vi "STAGE+mono+counter_edit3.vi"() -> ()   [LabVIEW 2017]
panel:
  out "XY Graph":cluster{"Y":dbl[], "Y":dbl[]}[](graph)
  in  "Integrating time, 10^-7 sec":dbl=10000000.0
  out "Timeout 2":bool
  in  "scan from":i32=2600
  in  "scan to":i32=4000
  in  "?":bool
  in  "Exit Labview":bool
  in  "step size":dbl=10.0 min=0.0
  in  "?":bool
  out "Spectrum":waveform(dbl)(graph)
  out "Counts":i32
  in  "value (0)":dbl=-9.0
  out "Current WL Wavelength  2":u16 caption="Current Wavelength"
  out "Grt# 2":u8=1 min=1 max=3 step=1
  out "Blaze (nm)":u32=300
  out "Groove/mm":u32=1200
  in  "?":bool
  in  "Channel B Input":u16(ring)=2 items=["Input 1"=1, "Input 2"=2]
  in  "Trigger mode":u16(ring) items=["10 MHz"=0, "Input 2"=2, "Input T"=3]
  out "Current WL Wavelength":u16 caption="Current Wavelength"
  in  "Integrating time, 10^-7 sec":dbl=10000000.0
  in  "gate A mode (CW:0)":i16(slide) scale=0.0..2.0 scale format="%.2f"
  in  "Channel A Input":u16(ring)=1 items=["10 MHz", "Input 1"]
  in  "Time between measurements\n at one point (s)/Dwell Time":dbl=0.002 min=0.002 max=60.0 step=0.001
  in  "Number of Measurements\n to take at one point/ Number of Periods":u16=1 min=1 max=2000 step=1
  in  "Count Mode":u16(ring) items=["A,B for Preset T", "A-B for Preset T", "A+B for Preset T", "A for Preset B"]
  in  "GPIB address":string="23"
  out "Timeout":bool
  out "Serial":u32=12345
  out "Grt#":u8=1 min=1 max=3 step=1
  out "Blaze (nm)":u32=300
  out "Groove/mm":u32=1200
  out "time delay":u32=450000 min=1
  out "Mono port":T1(ring)
  in  "Get position":bool
  out "Position status":dbl format="%.3f"
  in  "Target position":dbl format="%.3f"
  in  "Move":bool
  in  "Motor OFF":bool
  in  "Motor ON":bool
  in  "Step Size [um]":i32=10
  in  "Axis":i32=1
  in  "Rep Rate [Hz]":dbl=500.0
  out "Shots":dbl
  in  "Averaging Time [s]":dbl=0.1
  out "Current Point":i32
  out "Slide":i32(slide) scale=0.0..100.0
  out "Current Position [mm]":dbl
  in  "Axis initial position [mm]":dbl
  out "Axis final Position [mm]":dbl
  in  "Data Points (100 default)":i32=100
  in  "Collect Data!":bool
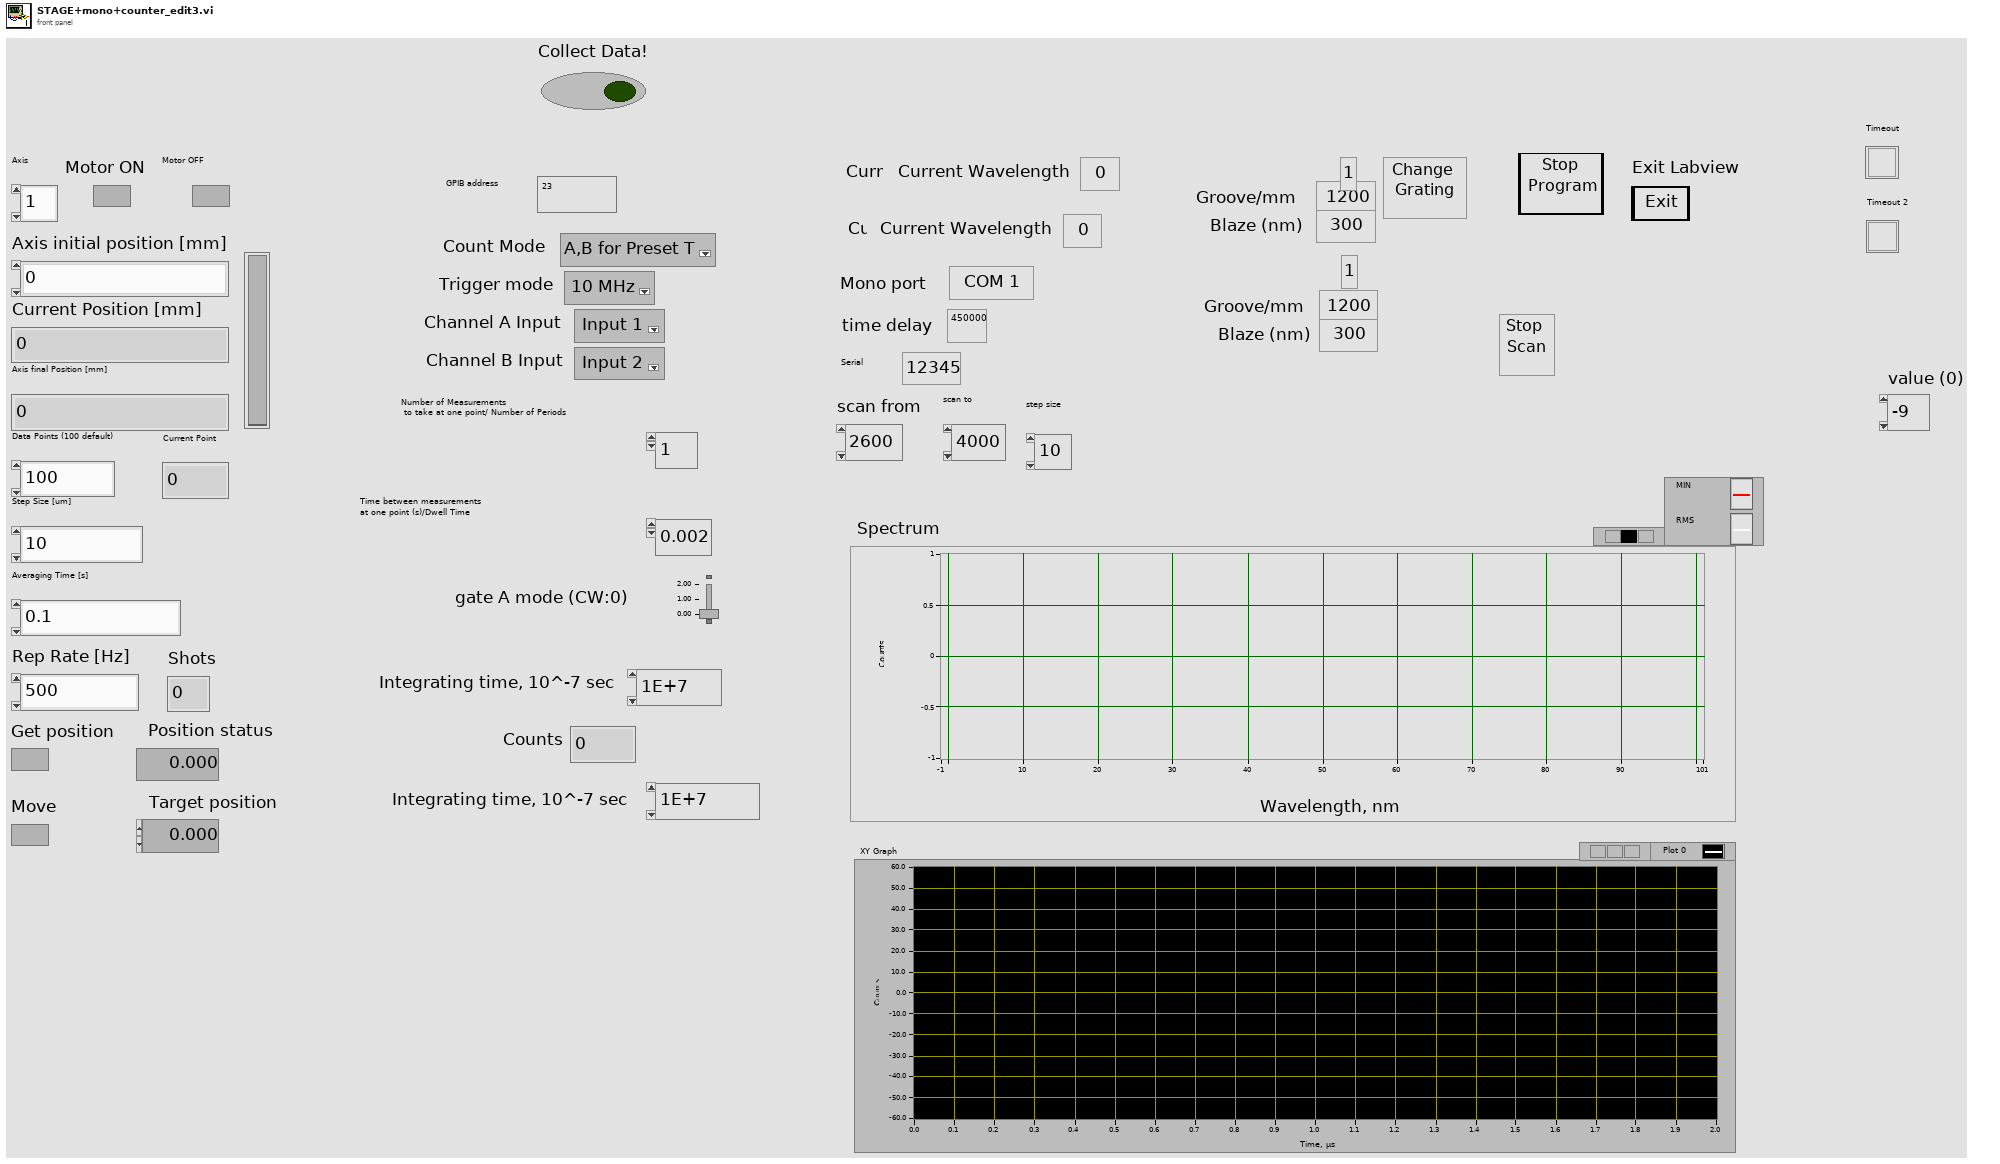
[diagram p1: front panel]
types:
  T1 = enum8{"COM 1", "COM 2", "COM 3", "COM 4", "COM 5", "COM 6", "COM 7", "COM 8", "COM 9"}
  T2 = cluster{"input XON/XOFF":bool, "input HW Handshake":bool, "input alt HW HShk":bool, "output XON/XOFF":bool, "output HW Handshake":bool, "output alt HW HShk":bool, "XOFF byte":u8, "XON byte":u8, "parity error byte":u16}
  T3 = enum16{"no parity", "odd parity", "even parity", "mark parity", "space parity"}
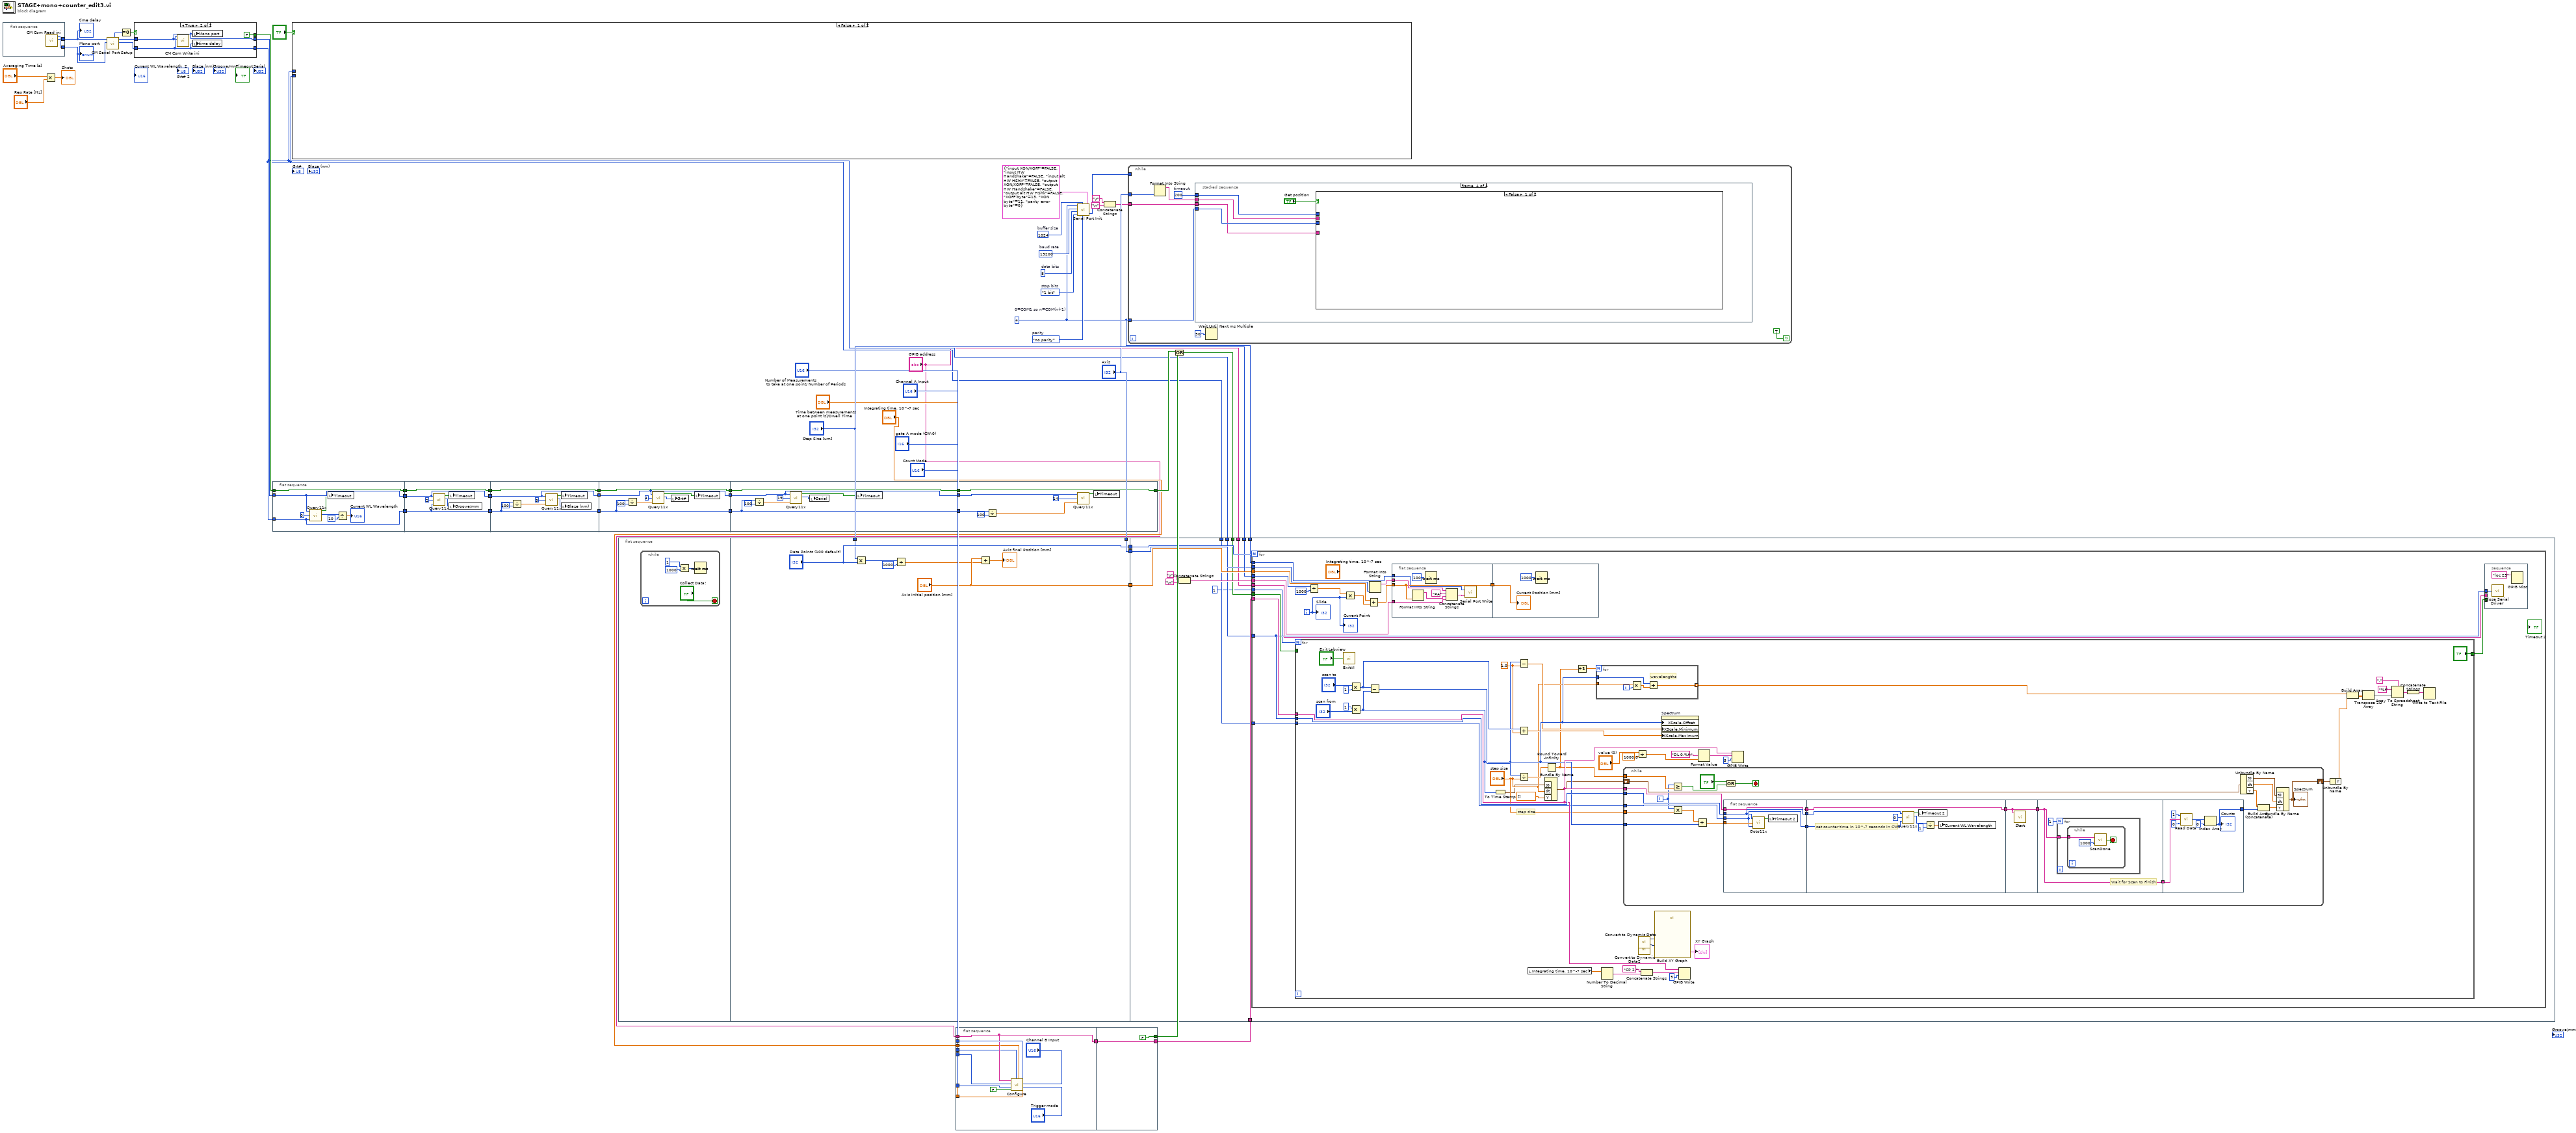
[diagram p0: block diagram]
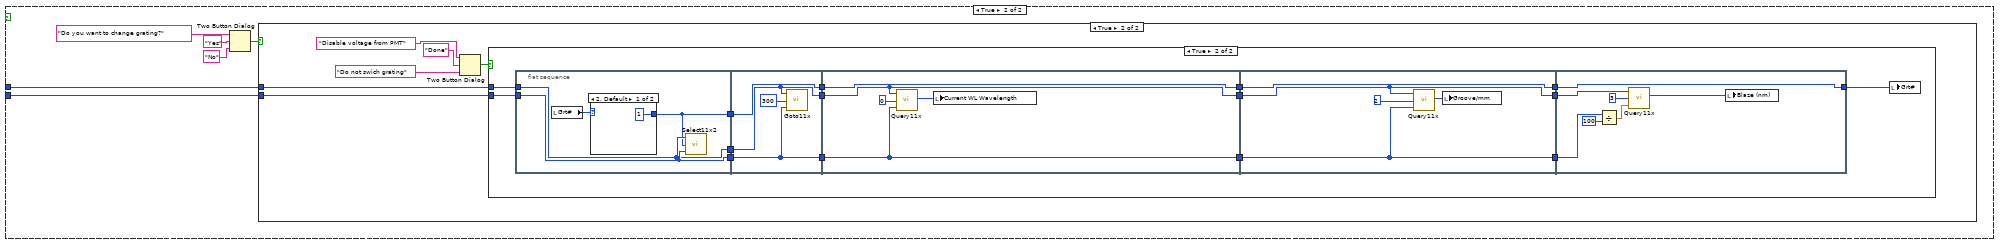
[diagram p2: hidden frame]
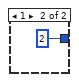
[diagram p5: hidden frame]
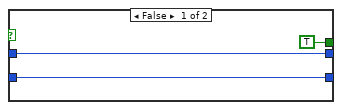
[diagram p6: hidden frame]
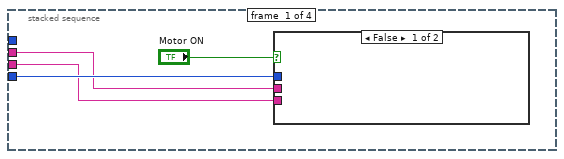
[diagram p7: hidden frame]
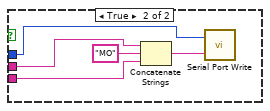
[diagram p8: hidden frame]
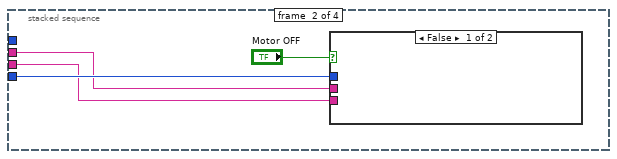
[diagram p9: hidden frame]
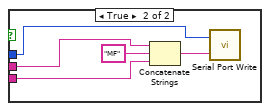
[diagram p10: hidden frame]
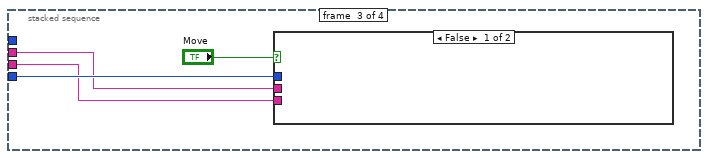
[diagram p11: hidden frame]
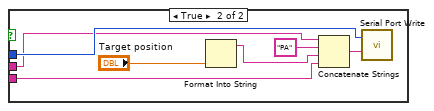
[diagram p12: hidden frame]
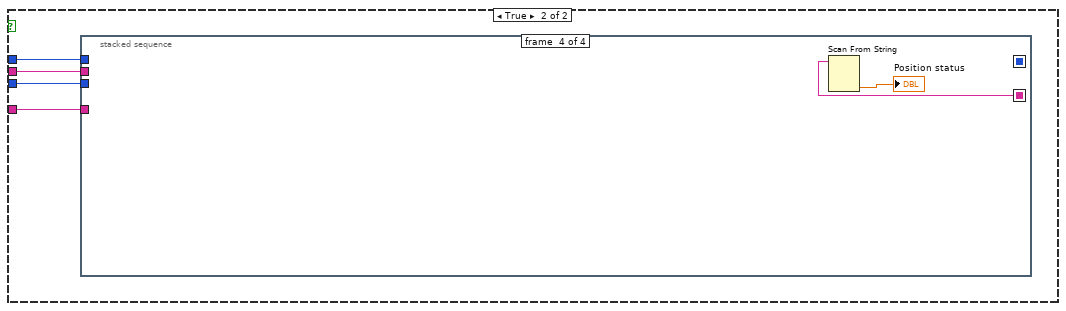
[diagram p13: hidden frame]
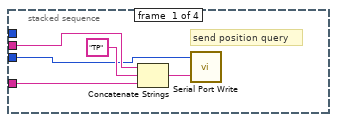
[diagram p14: hidden frame]
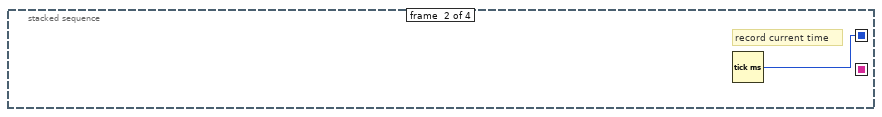
[diagram p15: hidden frame]
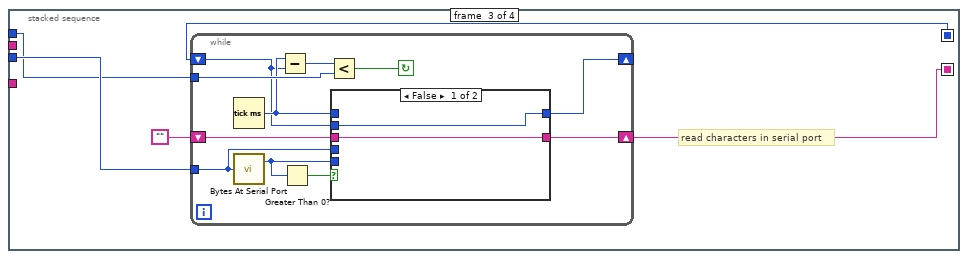
[diagram p16: hidden frame]
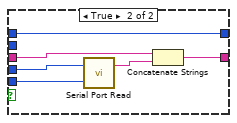
[diagram p17: hidden frame]
diagram:
  w46 = u32 19200  # baud rate
  w45 = u16 8  # data bits
  w44 = enum16{"1 bit", "1.5 bits", "2 bits"}."1 bit"  # stop bits
  w49 = T3."no parity"  # parity
  w43 = 4  # 0=COM1 so n=COM(n+1)
  w48 = u16 1024  # buffer size
  n1 = flat-sequence {
    tunnel: [w58] -> w21
    tunnel: [w57] -> w20
    frame #0 {
      n2 = call "CM Com Read ini.vi"() -> ("Mono port"=w57:T1, "time delay1"=w58:u32)  [unwired: 7 in]
    }
  }
  n3 = Multiply(x="Averaging Time [s]", y="Rep Rate [Hz]") -> (x*y=→"Shots":dbl)
  n4 = call "CM Serial Port Setup.vi"("COM port"=w20, "time delay"=w21) -> ("time delay1"=w16:u32, "DK port Out"=w17:T1, "error code"=w19:i32)  [unwired: 7 in]
  n5 = Equal To 0?(x=w19) -> (x = 0?=w18:bool)
  n6 = case shown="True" w18 {
    tunnel: w17 -> [w61 w64]
    tunnel: w16 -> [w60 w63]
    tunnel: [w61 w64] -> w3
    tunnel: [w60 w63] -> w2
    tunnel: [TRUE FALSE] -> w15
    frame False {
    }
    frame True {
      n7 = call "CM Com Write ini.vi"("time delay1"=w64, "Mono port"=w63) -> ()  [unwired: 7 in]
      n8 = local write "Mono port"(w64) -> ()
      n9 = local write "time delay"(w63) -> ()
    }
  }
  n10 = flat-sequence {
    tunnel: w2 -> [w70]
    tunnel: [w70] -> w37
    tunnel: w3 -> [w72]
    tunnel: [w72] -> w36
    tunnel: w15 -> [w68]
    tunnel: [w68] -> w35
    tunnel: w37 -> [w75]
    tunnel: [w75] -> w34
    tunnel: w36 -> [w77]
    tunnel: [w77] -> w33
    tunnel: w35 -> [w73]
    tunnel: [w73] -> w32
    tunnel: w34 -> [w85]
    tunnel: [w85] -> w31
    tunnel: w33 -> [w82]
    tunnel: [w82] -> w30
    tunnel: w32 -> [w79]
    tunnel: [w79] -> w29
    tunnel: w31 -> [w93]
    tunnel: [w93] -> w28
    tunnel: w30 -> [w90]
    tunnel: [w90] -> w27
    tunnel: w29 -> [w87]
    tunnel: [w87] -> w26
    tunnel: w28 -> [w101]
    tunnel: [w101] -> w25
    tunnel: w27 -> [w98]
    tunnel: [w98] -> w24
    tunnel: w26 -> [w95]
    tunnel: [w95] -> w23
    tunnel: w25 -> [w108]
    tunnel: w24 -> [w105]
    tunnel: [w103] -> w9
    tunnel: w23 -> [w103]
    frame #0 {
      n11 = call "Query11x.vi"("port number"=w72, "QUERY"=u16 0, "time delay"=w70) -> ("timeout"=w69:bool, "STATUS MESSAGE"=w67:u16)  [unwired: 2 out]
      n12 = local write "Timeout"(w69) -> ()
      n13 = Divide(x=w67, y=10 ("Numeric")) -> (x/y=→"Current WL Wavelength":dbl)
    }
    frame #1 {
      n14 = call "Query11x.vi"("port number"=w77, "QUERY"=u16 2, "time delay"=w75) -> ("timeout"=w74:bool, "STATUS MESSAGE"=w76:u16)  [unwired: 2 out]
      n15 = local write "Timeout"(w74) -> ()
      n16 = local write "Groove/mm"(w76) -> ()
    }
    frame #2 {
      n17 = Divide(x=w85, y=i16 100 ("device (1)")) -> (x/y=w83:dbl)
      n18 = call "Query11x.vi"("port number"=w82, "QUERY"=u16 3, "time delay"=w83) -> ("timeout"=w80:bool, "STATUS MESSAGE"=w81:u16)  [unwired: 2 out]
      n19 = local write "Timeout"(w80) -> ()
      n20 = local write "Blaze (nm)"(w81) -> ()
    }
    frame #3 {
      n21 = Divide(x=w93, y=i16 100 ("device (1)")) -> (x/y=w91:dbl)
      n22 = call "Query11x.vi"("port number"=w90, "QUERY"=u16 4, "time delay"=w91) -> ("timeout"=w88:bool, "STATUS MESSAGE"=w89:u16)  [unwired: 2 out]
      n23 = local write "Grt#"(w89) -> ()
      n24 = local write "Timeout"(w88) -> ()
    }
    frame #4 {
      n25 = Divide(x=w101, y=i16 100 ("device (1)")) -> (x/y=w99:dbl)
      n26 = call "Query11x.vi"("port number"=w98, "QUERY"=u16 19, "time delay"=w99) -> ("timeout"=w96:bool, "STATUS MESSAGE"=w97:u16)  [unwired: 2 out]
      n27 = local write "Serial"(w97) -> ()
      n28 = local write "Timeout"(w96) -> ()
    }
    frame #5 {
      n29 = Divide(x=w108, y=i16 100 ("device (1)")) -> (x/y=w106:dbl)
      n30 = call "Query11x.vi"("port number"=w105, "QUERY"=u16 14, "time delay"=w106) -> ("timeout"=w104:bool)  [unwired: 3 out]
      n31 = local write "Timeout"(w104) -> ()
    }
  }
  n32 = case shown="False" "?" {
    tunnel: w2 -> [_ w111]
    tunnel: w3 -> [_ w110]
    frame False {
    }
    frame True {
      n33 = Two Button Dialog(message="Do you want to change grating?", 1:"No" ("F button name (\"Cancel\")"), 2:"Yes" ("T button name (\"OK\")")) -> (T button?=w112:bool)
      n34 = case shown="True" w112 {
        tunnel: w111 -> [_ w117]
        tunnel: w110 -> [_ w116]
        frame False {
        }
        frame True {
          n35 = Two Button Dialog(message="Disable voltage from PMT", 1:"Do not swich grating" ("F button name (\"Cancel\")"), 2:"Done" ("T button name (\"OK\")")) -> (T button?=w118:bool)
          n36 = case shown="True" w118 {
            tunnel: w117 -> [_ w136]
            tunnel: w116 -> [_ w135]
            frame False {
            }
            frame True {
              n37 = flat-sequence {
                tunnel: w136 -> [w140]
                tunnel: [w140] -> w133
                tunnel: w135 -> [w139]
                tunnel: [w139] -> w132
                tunnel: [w137] -> w131
                tunnel: w133 -> [w144]
                tunnel: [w144] -> w130
                tunnel: w132 -> [w145]
                tunnel: [w145] -> w129
                tunnel: w131 -> [w143]
                tunnel: [w143] -> w128
                tunnel: w130 -> [w151]
                tunnel: [w151] -> w127
                tunnel: w129 -> [w150]
                tunnel: [w150] -> w126
                tunnel: w128 -> [w147]
                tunnel: [w147] -> w125
                tunnel: w127 -> [w154]
                tunnel: [w154] -> w124
                tunnel: w126 -> [w155]
                tunnel: [w155] -> w123
                tunnel: w125 -> [w152]
                tunnel: [w152] -> w122
                tunnel: w124 -> [w159]
                tunnel: w123 -> [w160]
                tunnel: [w157] -> w134
                tunnel: w122 -> [w157]
                frame #0 {
                  n38 = local read "Grt#"() -> (w138:u8)
                  n39 = case shown="2, Default" w138 {
                    tunnel: [1 2] -> w137
                    frame 2, Default {
                    }
                    frame 1 {
                    }
                  }
                  n40 = call "Select11x2.vi"("time delay"=w140, "NEW GRT?"=w137, "port number"=w139) -> ()  [unwired: 3 out]
                }
                frame #1 {
                  n41 = call "Goto11x.vi"("time delay"=w144, "WAVELENGTH"=u16 300, "port number"=w145) -> ()  [unwired: 3 out]
                }
                frame #2 {
                  n42 = call "Query11x.vi"("port number"=w150, "QUERY"=u16 0, "time delay"=w151) -> ("STATUS MESSAGE"=w148:u16)  [unwired: 3 out]
                  n43 = local write "Current WL Wavelength"(w148) -> ()
                }
                frame #3 {
                  n44 = call "Query11x.vi"("port number"=w155, "QUERY"=u16 2, "time delay"=w154) -> ("STATUS MESSAGE"=w153:u16)  [unwired: 3 out]
                  n45 = local write "Groove/mm"(w153) -> ()
                }
                frame #4 {
                  n46 = Divide(x=w159, y=i16 100 ("device (1)")) -> (x/y=w161:dbl)
                  n47 = call "Query11x.vi"("port number"=w160, "QUERY"=u16 3, "time delay"=w161) -> ("STATUS MESSAGE"=w158:u16)  [unwired: 3 out]
                  n48 = local write "Blaze (nm)"(w158) -> ()
                }
              }
              n49 = local write "Grt#"(w134) -> ()
            }
          }
        }
      }
    }
  }
  n50 = flat-sequence {
    tunnel: ["Data Points (100 default)"] -> w56
    tunnel: "Axis" -> [w175]
    tunnel: ["Axis initial position [mm]"] -> w55
    tunnel: "Step Size [um]" -> [w168]
    tunnel: [w175] -> w54
    tunnel: w56 -> [w189]
    tunnel: w55 -> [w188]
    tunnel: "Step Size [um]" -> [w187]
    tunnel: w54 -> [w186]
    tunnel: w43 -> [w182]
    tunnel: w5 -> [w181]
    tunnel: w4 -> [w180]
    tunnel: w3 -> [w179]
    tunnel: w2 -> [w178]
    tunnel: "GPIB address" -> [w177]
    frame #0 {
      n51 = while {
        stop <- "Collect Data!" stop-if-true
        n52 = Multiply(x=1, y=1000) -> (x*y=w167:i32)
        n53 = Wait (ms)(milliseconds to wait=w167) -> ()  [unwired: 1 out]
      }
    }
    frame #1 {
      n54 = Multiply(x=w168, y="Data Points (100 default)") -> (x*y=w171:i32)
      n55 = Divide(x=w171, y=1000) -> (x/y=w170:dbl)
      n56 = Add(x="Axis initial position [mm]", y=w170) -> (x+y=→"Axis final Position [mm]":dbl)
    }
    frame #2 {
      n57 = Concatenate Strings("\r", "\n") -> (w183:string)
      n58 = for {
        N: w189 -> [_]
        tunnel: w188 -> [w207]
        tunnel: w187 -> [w203]
        tunnel: w186 -> [w200]
        tunnel: w183 -> [w197]
        tunnel: w182 -> [w198]
        tunnel: w181 -> [w195]
        tunnel: w180 -> [w194]
        tunnel: w179 -> [w191]
        tunnel: w178 -> [w193]
        tunnel: w177 -> [w192]
        tunnel: 1 -> [w190]
        i -> [w208]
        n59 = for {
          N: w190 -> [_]
          tunnel: w191 -> [w250]
          tunnel: w193 -> [w242]
          tunnel: ["?"] -> w196
          tunnel: w194 -> [_]
          tunnel: w195 -> [w249]
          w239 = 1.0 ("x")
          # "step size"
          n60 = call "ExitVI.vi"("Exit Labview"="Exit Labview") -> ()
          n61 = Multiply(x="scan to", y=1) -> (x*y=w246:i32)
          n62 = Multiply(x=1, y="scan from") -> (x*y=w244:i32)
          n63 = Subtract(x=w246, y=w244) -> (x-y=w253:i32)
          n64 = To Time Stamp(1:w244) -> (0:w233:timestamp)
          n65 = Subtract(x=w244, y=w239) -> (x-y=w238:dbl)
          n66 = Add(x=w246, y=w239) -> (x+y=w240:dbl)
          n67 = Divide(x=w253, y="step size") -> (x/y=w241:dbl)
          n68 = local read "Integrating time, 10^-7 sec"() -> (w235:dbl)
          n69 = Bundle By Name("t0"=w233, "dt"="step size", "Y"=dbl[] []) -> (w232:waveform(dbl))  [unwired: 1 in]
          n70 = Round Toward -Infinity(1:w241) -> (0:w236:dbl)
          n71 = Increment(x=w236) -> (x+1=w231:dbl)
          n72 = for {
            N: w231 -> [_]
            tunnel: "step size" -> [w309]
            tunnel: w244 -> [w307]
            tunnel: [w305] -> w225 mode=indexing
            i -> [w308]
            # "wavelengths"
            n73 = Multiply(x=w309, y=w308) -> (x*y=w306:dbl)
            n74 = Add(x=w307, y=w306) -> (x+y=w305:dbl)
          }
          n75 = Number To Decimal String(number=w235) -> (decimal integer string=w229:string)  [unwired: 1 in]
          n76 = while {
            tunnel: w244 -> [w266]
            tunnel: "step size" -> [w278]
            tunnel: w250 -> [w276]
            tunnel: w242 -> [w275]
            tunnel: w236 -> [w274]
            shift-right: [w263] -> w218
            shift-left: w232 -> [w272]
            tunnel: w249 -> [w262]
            i -> [w269]
            stop <- w273 stop-if-true
            n77 = Greater Or Equal?(x=w269, y=w274) -> (x >= y?=w264:bool)
            n78 = Multiply(x=w269, y=w278) -> (x*y=w277:dbl)
            n79 = Add(x=w277, y=w266) -> (x+y=w254:dbl)
            n80 = flat-sequence {
              tunnel: w254 -> [w283]
              tunnel: w276 -> [w282]
              tunnel: [w282] -> w260
              tunnel: w275 -> [w281]
              tunnel: [w281] -> w259
              tunnel: w262 -> [w279]
              tunnel: [w279] -> w258
              tunnel: w260 -> [w290]
              tunnel: w259 -> [w289]
              tunnel: w258 -> [w287]
              tunnel: [w287] -> w257
              tunnel: w257 -> [w292]
              tunnel: [w292] -> w256
              tunnel: w256 -> [w293]
              tunnel: [w293] -> w255
              tunnel: w255 -> [w300]
              tunnel: [w299] -> w261
              frame #0 {
                n81 = call "Goto11x.vi"("time delay"=w281, "WAVELENGTH"=w283, "port number"=w282) -> ("timeout"=w280:bool)  [unwired: 2 out]
                n82 = local write "Timeout 2"(w280) -> ()
              }
              frame #1 {
                # "set counter time in 10^-7 seconds in CW"
                n83 = call "Query11x.vi"("port number"=w290, "QUERY"=0, "time delay"=w289) -> ("timeout"=w288:bool, "STATUS MESSAGE"=w286:u16)  [unwired: 2 out]
                n84 = local write "Timeout 2"(w288) -> ()
                n85 = Divide(x=w286, y=1) -> (x/y=w285:dbl)
                n86 = local write "Current WL Wavelength"(w285) -> ()
              }
              frame #2 {
                n87 = call "Start.vi"("GPIB Address"=w292) -> ()  [unwired: 9 in]
              }
              frame #3 {
                # "Wait for Scan to Finish"
                n88 = for {
                  N: 1 -> [_]
                  tunnel: w293 -> [w295]
                  n89 = while {
                    tunnel: w295 -> [w296]
                    stop <- w298 stop-if-true
                    n90 = call "ScanDone.vi"("Wait (ms)"=1000, "GPIB Address"=w296) -> ("Scan Finished?"=w298:bool)
                  }
                }
              }
              frame #4 {
                n91 = call "Read Data.vi"("Channel Number"=0, "GPIB Address"=w300, "Number of Datapoints"=1) -> ("Data"=w301:i32[])
                n92 = Index Array(array=w301, index=0) -> (element=w299:i32)
                "Counts" <- w299
              }
            }
            n93 = Or(x="?", y=w264) -> (x .or. y?=w273:bool)
            n94 = Unbundle By Name(w272) -> ("t0"=w270:timestamp, "dt"=w271:dbl, "Y"=w268:dbl[])
            n95 = Build Array (concatenate)(w268, w261) -> (w267:dbl[])
            n96 = Bundle By Name("t0"=w270, "dt"=w271, "Y"=w267) -> (w263:waveform(dbl))  [unwired: 1 in]
            "Spectrum" <- w263
          }
          n97 = Divide(x="value (0)", y=1000.0) -> (x/y=w212:dbl)
          n98 = call "Convert to Dynamic Data"() -> ("Dynamic Data Type"=w209:dynamicdata)  [unwired: 4 in]
          n99 = call "Convert to Dynamic Data2"() -> ("Dynamic Data Type"=w210:dynamicdata)  [unwired: 4 in]
          n100 = Concatenate Strings("CP 2,", w229) -> (w227:string)
          n101 = call "Build XY Graph"("Y Input"=w210, "X Input"=w209) -> ("XY Graph"=→"XY Graph":cluster{"Y":dbl[], "Y":dbl[]}[])  [unwired: 3 in, 6 out]
          n102 = property on="Spectrum" class="WFGraph (strict)"("XScale.Offset"=w244, "XScale.Minimum"=w238, "XScale.Maximum"=w240) -> ()  [unwired: 2 in, 2 out]
          n103 = GPIB Write(0:w249, 1:w227, 2:i16 5 ("mode (0)")) -> ()  [unwired: 2 in, 2 out]
          n104 = Format Value(format string="DL 0,%f;", value (0)=w212) -> (output string=w216:string)  [unwired: 1 in]
          n105 = GPIB Write(0:w249, 1:w216, 2:i16 5 ("mode (0)")) -> ()  [unwired: 2 in, 2 out]
          n106 = Unbundle By Name(w218) -> ("Y"=w226:dbl[])
          n107 = Build Array(w225, w226) -> (w220:dbl[][])
          n108 = Transpose 2D Array(2D array=w220) -> (transposed array=w219:dbl[][])
          n109 = Array To Spreadsheet String(delimiter (Tab)=",", array=w219, 3:"%f" ("format string")) -> (spreadsheet string=w221:string)
          n110 = Concatenate Strings(w221) -> (w222:string)
          n111 = Write to Text File(text=w222) -> ()  [unwired: 3 in, 3 out]
        }
        n112 = Divide(x=w203, y=1000) -> (x/y=w202:dbl)
        n113 = Multiply(x=w202, y=w208) -> (x*y=w206:dbl)
        n114 = Add(x=w207, y=w206) -> (x+y=w205:dbl)
        n115 = Format Into String(w200) -> (resulting string=w199:string)  [unwired: 3 in, 1 out]
        n116 = flat-sequence {
          tunnel: w205 -> [w314]
          tunnel: [w314] -> w201
          tunnel: w197 -> [w316]
          tunnel: w199 -> [w315]
          tunnel: w198 -> [w312]
          tunnel: w201 -> [w320]
          frame #0 {
            n117 = Format Into String(w314) -> (resulting string=w313:string)  [unwired: 3 in, 1 out]
            n118 = Wait (ms)(milliseconds to wait=u32 100) -> ()  [unwired: 1 out]
            n119 = Concatenate Strings(w315, "PA" ("Substring"), w313, w316) -> (w318:string)
            n120 = call <vilib>:"Serial Port Write.vi"("string to write"=w318, "port number"=w312) -> ()  [unwired: 1 out]
          }
          frame #1 {
            n121 = Wait (ms)(milliseconds to wait=u32 1000) -> ()  [unwired: 1 out]
            "Current Position [mm]" <- w320
          }
        }
        n122 = stacked-sequence {
          tunnel: w196 -> [_]
          tunnel: w191 -> [w311]
          tunnel: w192 -> [_]
          frame #0 {
            n123 = call <vilib>:"Close Serial Driver.vi"("port number"=w311) -> ()  [unwired: 1 out]
            n124 = GPIB Misc(0:"loc 23" ("command string")) -> ()  [unwired: 1 in, 3 out]
          }
        }
        "Current Point" <- w208
        "Slide" <- w208
      }
    }
  }
  n125 = flat-sequence {
    tunnel: "GPIB address" -> [w329]
    tunnel: [w329] -> w22
    tunnel: "Count Mode" -> [w330]
    tunnel: "Number of Measurements\n to take at one point/ Number of Periods" -> [w327]
    tunnel: "Time between measurements\n at one point (s)/Dwell Time" -> [w326]
    tunnel: "Channel A Input" -> [w331]
    tunnel: "gate A mode (CW:0)" -> [w323]
    tunnel: "Integrating time, 10^-7 sec" -> [w322]
    tunnel: w22 -> [w332]
    tunnel: [w332] -> w5
    tunnel: [FALSE] -> w10
    frame #0 {
      n126 = call "Configure.vi"("Dwell Time (s)"=w326, "Channel T Input"="Trigger mode", "Channel B Input"="Channel B Input", "Channel A Input"=w331, "Integrating time, 10^-7 sec"=w322, "gate mode (CW:0)"=w323, "Scan End Mode"=FALSE, "Number of Periods"=w327, "Count Mode"=w330, "GPIB Address"=w329) -> ()
    }
    frame #1 {
    }
  }
  n127 = call <vilib>:"Serial Port Init.vi"("flow control etc."=T2 {"input XON/XOFF"=FALSE, "input HW Handshake"=FALSE, "input alt HW HShk"=FALSE, "output XON/XOFF"=FALSE, "output HW Handshake"=FALSE, "output alt HW HShk"=FALSE, "XOFF byte"=13, "XON byte"=11, "parity error byte"=0}, "parity"=w49, "buffer size"=w48, "stop bits"=w44, "data bits"=w45, "baud rate"=w46, "port number"=w43) -> ("error code"=w42:i32)
  n128 = Concatenate Strings("\r", "\n") -> (w38:string)
  n129 = while {
    tunnel: w43 -> [w336]
    tunnel: w38 -> [w337]
    tunnel: w42 -> [_]
    tunnel: "Axis" -> [w334]
    stop <- TRUE continue-if-true
    w335 = u32 200  # timeout
    n130 = Format Into String(w334) -> (resulting string=w338:string)  [unwired: 3 in, 1 out]
    n131 = stacked-sequence {
      tunnel: w338 -> [w342 w352 w361 w373]
      tunnel: w337 -> [w341 w351 w360 w370]
      tunnel: w336 -> [w343 w353 w362 w372]
      tunnel: w335 -> [_ _ _ w371]
      frame #0 {
        n132 = case shown="False" "Motor ON" {
          tunnel: w343 -> [_ w349]
          tunnel: w342 -> [_ w346]
          tunnel: w341 -> [_ w345]
          frame False {
          }
          frame True {
            n133 = Concatenate Strings(w346, "MO" ("Substring"), w345) -> (w347:string)
            n134 = call <vilib>:"Serial Port Write.vi"("string to write"=w347, "port number"=w349) -> ()  [unwired: 1 out]
          }
        }
      }
      frame #1 {
        n135 = case shown="False" "Motor OFF" {
          tunnel: w353 -> [_ w358]
          tunnel: w352 -> [_ w355]
          tunnel: w351 -> [_ w354]
          frame False {
          }
          frame True {
            n136 = Concatenate Strings(w355, "MF" ("Substring"), w354) -> (w356:string)
            n137 = call <vilib>:"Serial Port Write.vi"("string to write"=w356, "port number"=w358) -> ()  [unwired: 1 out]
          }
        }
      }
      frame #2 {
        n138 = case shown="False" "Move" {
          tunnel: w362 -> [_ w369]
          tunnel: w361 -> [_ w366]
          tunnel: w360 -> [_ w365]
          frame False {
          }
          frame True {
            n139 = Format Into String("Target position") -> (resulting string=w363:string)  [unwired: 3 in, 1 out]
            n140 = Concatenate Strings(w366, "PA" ("Substring"), w363, w365) -> (w367:string)
            n141 = call <vilib>:"Serial Port Write.vi"("string to write"=w367, "port number"=w369) -> ()  [unwired: 1 out]
          }
        }
      }
      frame #3 {
        n142 = case shown="False" "Get position" {
          tunnel: w373 -> [_ w378]
          tunnel: w372 -> [_ w377]
          tunnel: w371 -> [_ w376]
          tunnel: w370 -> [_ w375]
          frame False {
          }
          frame True {
            n143 = stacked-sequence {
              seq-local: [_ w384 _ _] -> [_ _ w386 _]
              seq-local: [_ _ w385 _] -> [_ _ _ w410]
              tunnel: w378 -> [w381 _ _ _]
              tunnel: w377 -> [w380 _ w389 _]
              tunnel: w376 -> [_ _ w387 _]
              tunnel: w375 -> [w379 _ _ _]
              frame #0 {
                # "send position query"
                n144 = Concatenate Strings(w381, "TP" ("Substring"), w379) -> (w382:string)
                n145 = call <vilib>:"Serial Port Write.vi"("string to write"=w382, "port number"=w380) -> ()  [unwired: 1 out]
              }
              frame #1 {
                # "record current time"
                n146 = Tick Count (ms)() -> (millisecond timer value=w384:u32)
              }
              frame #2 {
                # "read characters in serial port"
                n147 = while {
                  shift-left: w386 -> [w390]
                  shift-right: [w391] -> _
                  tunnel: w387 -> [w394]
                  shift-left: "" -> [w397]
                  shift-right: [w396] -> w385
                  tunnel: w389 -> [w398]
                  stop <- w393 continue-if-true
                  n148 = Tick Count (ms)() -> (millisecond timer value=w392:u32)
                  n149 = call <vilib>:"Bytes At Serial Port.vi"("port number"=w398) -> ("byte count"=w399:u32)  [unwired: 1 out]
                  n150 = Subtract(x=w392, y=w390) -> (x-y=w395:u32)
                  n151 = Greater Than 0?(x=w399) -> (x > 0?=w400:bool)
                  n152 = Less?(x=w395, y=w394) -> (x < y?=w393:bool)
                  n153 = case shown="False" w400 {
                    tunnel: w399 -> [_ w408]
                    tunnel: w398 -> [_ w407]
                    tunnel: w397 -> [w402 w405]
                    tunnel: [w402 w404] -> w396
                    tunnel: [w401 w403] -> w391
                    tunnel: w392 -> [_ w403]
                    tunnel: w390 -> [w401 _]
                    frame False {
                    }
                    frame True {
                      n154 = call <vilib>:"Serial Port Read.vi"("requested byte count"=w408, "port number"=w407) -> ("string read"=w406:string)  [unwired: 1 out]
                      n155 = Concatenate Strings(w405, w406) -> (w404:string)
                    }
                  }
                }
              }
              frame #3 {
                n156 = Scan From String(input string=w410) -> (output 1=→"Position status":dbl)  [unwired: 4 in, 3 out]
              }
            }
          }
        }
      }
    }
    n157 = Wait Until Next ms Multiple(millisecond multiple=u32 50) -> ()  [unwired: 1 out]
  }
  n158 = Or(x=w9, y=w10) -> (x .or. y?=w4:bool)
  "Mono port" <- w20
  "time delay" <- w21
